vi "Configure UI Dialog.vi"(8 "error in (no error)":errorcluster, 11 "Str Refnum":refnum<vi>) -> (0 "Error out":errorcluster)   [LabVIEW 2023, in "VeriStand Console.lvlib"]
uses:
  VeriStand Console.lvlib
  <vilib>/registry/registry.llb/Registry RtKey.ctl
  <vilib>/registry/registry.llb/Registry SAM.ctl
panel:
  in  "OK":bool
  in  "Background Color":u32(colorbox)
  in  "Text Color":u32(colorbox)
  in  "Size":string(combo)
  in  "Font":string(combo)
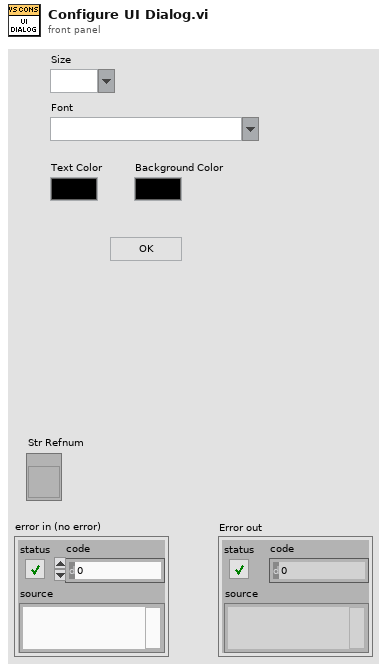
[diagram p1: front panel]
types:
  T1 = typedef "Registry SAM.ctl" = enum32{"KEY_QUERY_VALUE", "KEY_SET_VALUE", "KEY_CREATE_SUB_KEY", "KEY_ENUMERATE_SUB_KEYS", "KEY_NOTIFY", "KEY_CREATE_LINK", "KEY_READ", "KEY_WRITE", "KEY_ALL_ACCESS", "KEY_READ | KEY_WRITE"}
  T2 = typedef "Registry RtKey.ctl" = enum32{"HKEY_CLASSES_ROOT", "HKEY_CURRENT_USER", "HKEY_LOCAL_MACHINE", "HKEY_USERS", "HKEY_PERFORMANCE_DATA", "HKEY_CURRENT_CONFIG", "HKEY_DYN_DATA"}
  T3 = typedef "Registry refnum.ctl" = refnum<k1>
  T4 = cluster{"numValues":i32, "maxValueNameLen":i32, "maxValueDataLen":i32}
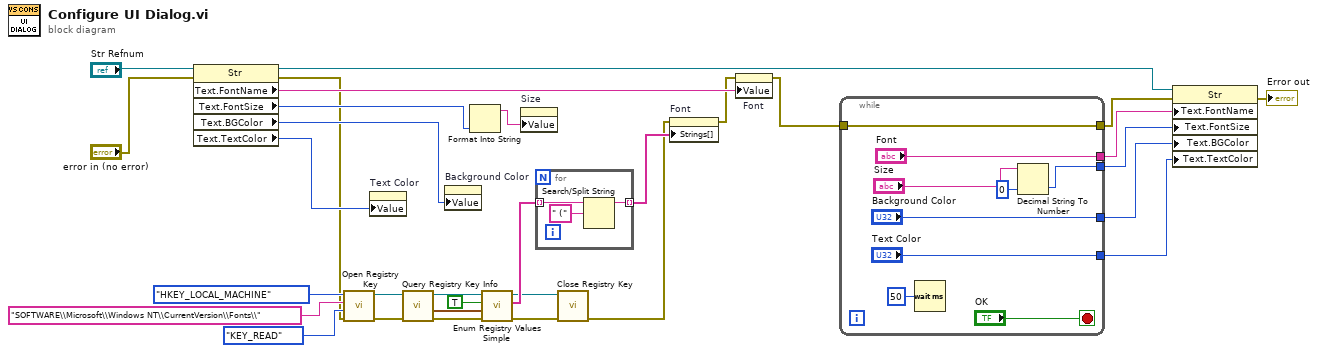
[diagram p0: block diagram]
diagram:
  n1 = property class="Str"(reference="Str Refnum", error in="error in (no error)") -> (reference out=w5:refnum<vi>, error out=w1:errorcluster, "Text.FontName"=w14:string, "Text.FontSize"=w18:u32, "Text.BGColor"=w15:u32, "Text.TextColor"=w16:u32)
  n2 = call <vilib>:"Open Registry Key.vi"("error in (no error)"=w1, "security access mask (KEY_READ | KEY_WRITE)"=Registry_SAM."KEY_READ", "subkey"="SOFTWARE\\Microsoft\\Windows NT\\CurrentVersion\\Fonts\\", "root key (HKEY_LOCAL_MACHINE)"=Registry_RtKey."HKEY_LOCAL_MACHINE") -> ("error out"=w23:errorcluster, "refnum out"=w22:T3)  [unwired: 6 in]
  n3 = property on="Text Color" class="ColBox"("Value"=w16) -> ()  [unwired: 2 in, 2 out]
  n4 = call <vilib>:"Query Registry Key Info.vi"("error in (no error)"=w23, "refnum"=w22) -> ("error out"=w26:errorcluster, "value info"=w29:T4, "refnum out"=w25:T3)  [unwired: 5 in, 2 out]
  n5 = property on="Background Color" class="ColBox"("Value"=w15) -> ()  [unwired: 2 in, 2 out]
  n6 = Format Into String(w18) -> (resulting string=w17:string)  [unwired: 3 in, 1 out]
  n7 = call <vilib>:"Enum Registry Values Simple.vi"("error in (no error)"=w26, "value info"=w29, "retrieve data? (F)"=TRUE, "refnum"=w25) -> ("error out"=w27:errorcluster, "values"=w31:string[], "refnum out"=w28:T3)  [unwired: 2 in, 3 out]
  n8 = property on="Size" class="CmbBox"("Value"=w17) -> ()  [unwired: 2 in, 2 out]
  n9 = for {
    tunnel: w31 -> [w34] mode=indexing
    tunnel: [w32] -> w13 mode=indexing
    n10 = Search/Split String(string=w34, search string/char (-)=" (") -> (substring before match=w32:string)  [unwired: 1 in, 2 out]
  }
  n11 = call <vilib>:"Close Registry Key.vi"("error in (no error)"=w27, "refnum"=w28) -> ("error out"=w10:errorcluster)  [unwired: 5 in]
  n12 = property on="Font" class="CmbBox"(error in=w10, "Strings[]"=w13) -> (error out=w12:errorcluster)  [unwired: 1 in, 1 out]
  n13 = property on="Font" class="CmbBox"(error in=w12, "Value"=w14) -> (error out=w11:errorcluster)  [unwired: 1 in, 1 out]
  n14 = while {
    tunnel: w11 -> [w35]
    tunnel: ["Text Color"] -> w9
    tunnel: ["Background Color"] -> w8
    tunnel: [w37] -> w7
    tunnel: ["Font"] -> w6
    tunnel: [w35] -> w4
    stop <- "OK" stop-if-true
    n15 = Wait (ms)(milliseconds to wait=u32 50) -> ()  [unwired: 1 out]
    n16 = Decimal String To Number(string="Size", default (0L)=u32 0 ("default (0 I32)")) -> (number=w37:u32)  [unwired: 1 in, 1 out]
  }
  n17 = property class="Str"(reference=w5, error in=w4, "Text.FontName"=w6, "Text.FontSize"=w7, "Text.BGColor"=w8, "Text.TextColor"=w9) -> (error out=→"Error out":errorcluster)  [unwired: 1 out]
